vi "Panel.vi"(11 "TipPanelExample in":refnum<class "TipPanelExample.lvclass">) -> ()   [LabVIEW 2021, in "TipStripOOPanelExample.lvlib" / "TipPanelExample.lvclass"]
uses:
  TipPanelExample.lvclass
  C:/GIT checkouts/TipStrip-OOPanel/Source/Classes/TipPanel/TipPanel.lvclass
  C:/Program Files/National Instruments/LabVIEW 2021/vi.lib/IlluminatedG/IG OOPanel/OOPanel/Panel/Panel.lvclass
  Classes/TipPanel/TipPanel.lvclass/TipPanel.ctl
  TipPanelExample.lvclass/TipPanelExample.ctl
  Classes/TipPanel/Read New Panel UE.vi
  <vilib>/Futures/Futures/Promise/Promise.lvclass
  <vilib>/IlluminatedG/IG OOPanel/OOPanel/Panel/Panel.lvclass
  <vilib>/IlluminatedG/IG OOPanel/OOPanel/OOPanel.lvlib
  Classes/TipPanel/TipPanel.lvclass
panel:
  out "current time":timestamp
  out "MyData":string
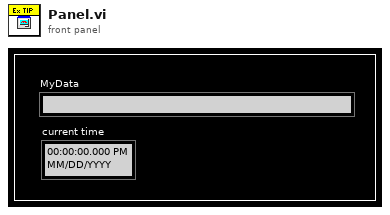
[diagram p1: front panel]
types:
  T1 = typedef "LVBoundsTypeDef.ctl" = cluster{"Width":u32, "Height":u32}
  T2 = typedef "OOPanel.lvlib/Panel.lvclass/Panel Events.ctl" = cluster{"Visbility":refnum<user-event>, "Close":refnum<user-event>}
  T3 = typedef "OOPanel.lvlib/Visibility State.ctl" = enum16{"Idle", "Closed", "Hidden", "Visible", "Subpanel", "Hidden Subpanel"}
  T4 = typedef "TipStripOOPanel.lvlib/TipPanel.lvclass/ToPanelUE.ctl" = cluster{"TipPanel":refnum<class>, "Promise.Size":refnum<class "Promise.lvclass">}
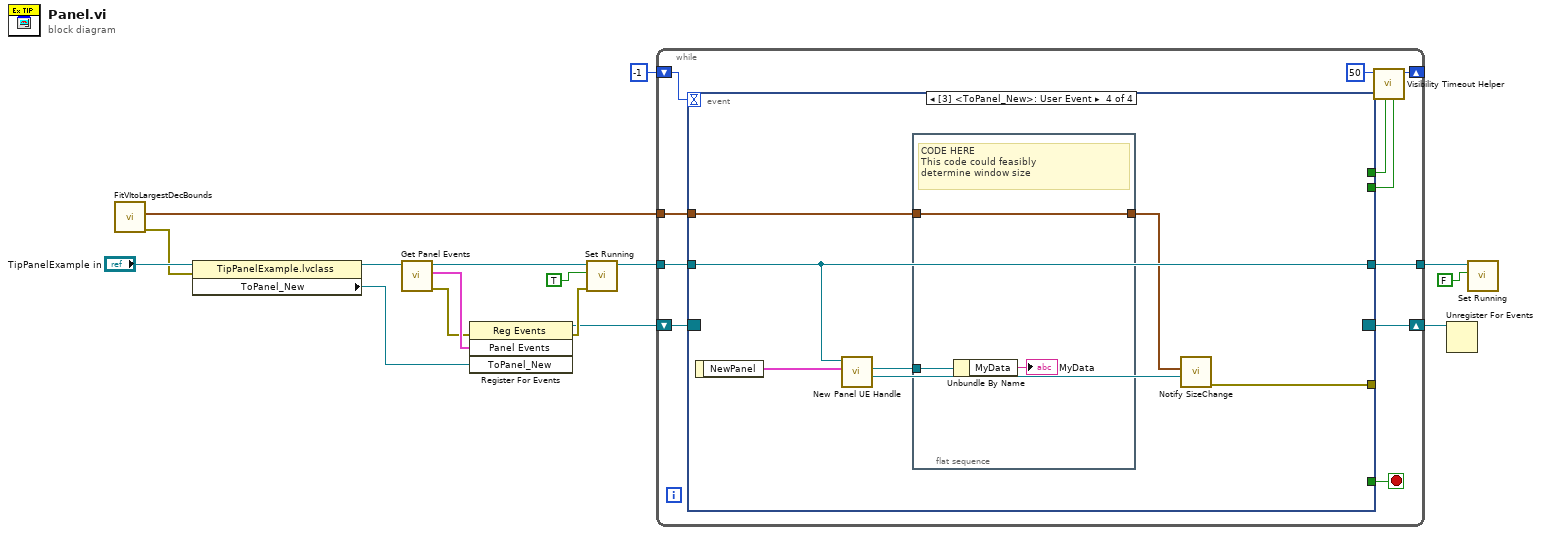
[diagram p0: block diagram]
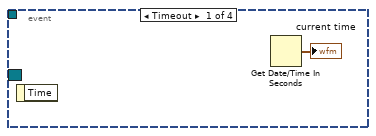
[diagram p2: hidden frame]
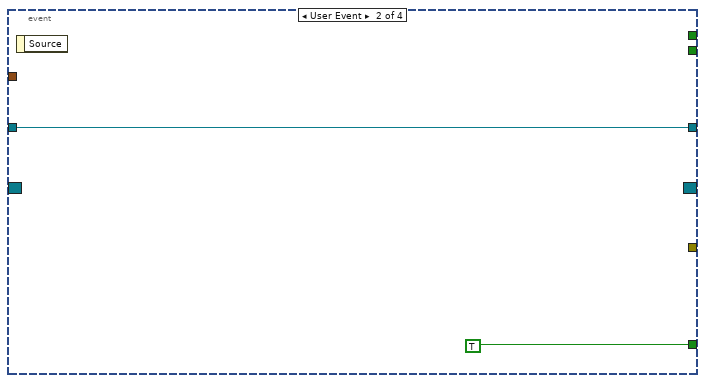
[diagram p3: hidden frame]
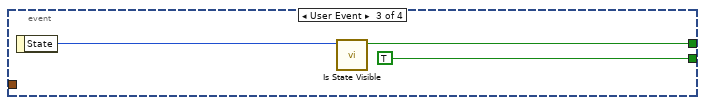
[diagram p4: hidden frame]
diagram:
  n1 = call "FitVItoLargestDecBounds.vi"() -> ("error out"=w1:errorcluster, "content size"=w3:T1)  [unwired: 9 in, 1 out]
  n2 = property class="TipPanelExample.lvclass"(reference="TipPanelExample in", error in=w1) -> (reference out=w5:refnum<class "TipPanelExample.lvclass">, "ToPanel_New"=w2:refnum<user-event>)  [unwired: 1 out]
  n3 = call <vilib>:"Get Panel Events.vi"("Panel in"=w5) -> ("error out"=w6:errorcluster, "Panel Events"=w16:T2, "Panel out"=w15:refnum<class "TipPanelExample.lvclass">)  [unwired: 8 in]
  n4 = register-events(error in=w6, w16, w2) -> (reference out=w12:refnum<event-registration>, error out=w13:errorcluster)  [unwired: 1 in]
  n5 = call <vilib>:"Set Running.vi"("error in (no error)"=w13, "Running"=TRUE, "Panel in"=w15) -> ("Panel out"=w11:refnum<class "TipPanelExample.lvclass">)  [unwired: 7 in, 1 out]
  n6 = while {
    shift-right: [w23] -> w8
    shift-left: w12 -> [w24]
    shift-right: [w26] -> _
    shift-left: -1 ("Timeout") -> [w25]
    tunnel: w11 -> [w19]
    tunnel: [w18] -> w7
    tunnel: w3 -> [w17]
    stop <- w20 stop-if-true
    n7 = event shown="[3] <ToPanel_New>: User Event" {
      selector: w24 -> [_ _ _ _]
      dyn-events: [_ _ _ _] -> w23
      timeout: w25 -> [_ _ _ _]
      tunnel: [_ _ w32 _] -> w22
      tunnel: [_ _ TRUE _] -> w21
      tunnel: [_ TRUE _ _] -> w20
      tunnel: w19 -> [_ w29 _ w40]
      tunnel: [_ w29 _ w40] -> w18
      tunnel: [_ _ _ w39] -> _
      tunnel: w17 -> [_ _ _ w36]
      event Timeout {
        n8 = event-data() -> ()  [unwired: 1 in, 1 out]
        n9 = Get Date/Time In Seconds() -> (seconds since 1Jan1904=→"current time":timestamp)
      }
      event User Event {
        n10 = event-data() -> ()  [unwired: 1 in, 1 out]
      }
      event User Event {
        n11 = event-data() -> ("State"=w33:T3)  [unwired: 1 in]
        n12 = call <vilib>:"Is State Visible.vi"("Visibility"=w33) -> ("Visible"=w32:bool)  [unwired: 10 in]
      }
      event User Event {
        n13 = event-data() -> ("NewPanel"=w34:T4)  [unwired: 1 in]
        n14 = call "New Panel UE Handle.vi"("NewPanel"=w34, "TipPanel in"=w40) -> ("Promise.Size"=w38:refnum<class "Promise.lvclass">, "DATA ONLY"=w35:refnum<class "TipPanelExample.lvclass">)  [unwired: 7 in, 1 out]
        n15 = flat-sequence {
          tunnel: [w43] -> w37
          tunnel: w36 -> [w43]
          tunnel: w35 -> [w42]
          frame #0 {
            # "CODE HERE\nThis code could feasibly\ndetermine window size"
            n16 = Unbundle By Name(w42) -> ("MyData"=→"MyData":string)
          }
        }
        n17 = call "Notify SizeChange.vi"("Promise in"=w38, "content size"=w37) -> ("error out"=w39:errorcluster)  [unwired: 9 in]
      }
    }
    n18 = call <vilib>:"Visibility Timeout Helper.vi"("Update?"=w21, "Use Timeout?"=w22, "Visible Timeout mS"=50) -> ("Timeout"=w26:i32)  [unwired: 8 in]
  }
  n19 = Unregister For Events(event registration refnum=w8) -> ()  [unwired: 1 in, 1 out]
  n20 = call <vilib>:"Set Running.vi"("Running"=FALSE, "Panel in"=w7) -> ()  [unwired: 8 in, 2 out]
